vi "cblas ztrsm.vi"(0 "A":T2, 1 "x":T2, 3 "alpha":cdb=1.0+0.0i, 5 "order":T5=101 items=["CblasRowMajor"=101, "CblasColMajor"=102], 6 "transA":T6=111 items=["CblasNoTrans"=111, "CblasTrans"=112, "CblasConjTrans "=113], 7 "uplo":T4=121 items=["CblasUpper"=121, "CblasLower"=122], 8 "lda":i32, 9 "m":i32=-1, 10 "ldx":i32, 11 "n":i32=-1, 12 "diag":T3=131 items=["CblasNonUnit"=131, "CblasUnit"=132], 13 "side":T1=141 items=["CblasLeft"=141, "CblasRight"=142]) -> (14 "ztrsm":T2, 19 "error":i32)   [LabVIEW 2017, in "NI_AALBLAS.lvlib"]
doc: "Operates on matrix <B>A</B> using the operation you select and solves one of the following linear equations for <B>trsm</B>: op(<B>A</B>)*<B>trsm</B> = <B>alpha</B>*<B>X</B> or <B>trsm</B>*op(<B>A</B>) = <B>alpha</B>*<B>X</B>. The data types you wire to <B>A</B> and <B>X</B> determine the polymorphic instance to use."
uses:
  <vilib>/Analysis/NI_AALBLAS.lvlib
  <vilib>/Analysis/Matrix/Datatypes/ComplexMatrix.ctl
  <vilib>/Analysis/BLAS.llb/Operation_Transpose.ctl
  <vilib>/Analysis/BLAS.llb/Order.ctl
  <vilib>/Analysis/BLAS.llb/UpLo.ctl
  <vilib>/Analysis/BLAS.llb/Diag.ctl
  <vilib>/Analysis/BLAS.llb/Side.ctl
  <resource>/lvblas.dll
  <vilib>/Analysis/Matrix/NI_Matrix.lvlib
panel:
  # "void cblas_ztrsm(order, side, uplo, transA, diag, m, n, *alpha, *A, lda, *X, ldx)"
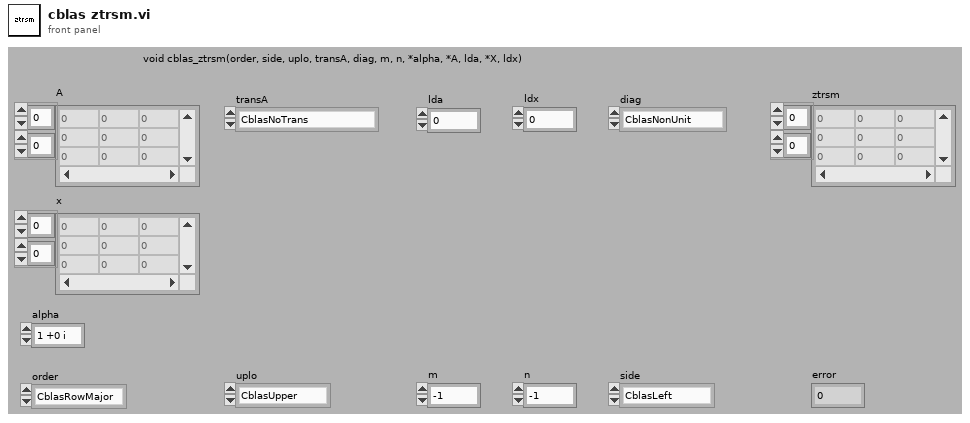
[diagram p1: front panel]
types:
  T1 = typedef "NI_AALBLAS.lvlib/Side.ctl" = i32
  T2 = typedef "NI_Matrix.lvlib/ComplexMatrix.ctl" = cdb[][]
  T3 = typedef "NI_AALBLAS.lvlib/Diag.ctl" = i32
  T4 = typedef "NI_AALBLAS.lvlib/UpLo.ctl" = i32
  T5 = typedef "NI_AALBLAS.lvlib/Order.ctl" = i32
  T6 = typedef "NI_AALBLAS.lvlib/Operation_Transpose.ctl" = i32
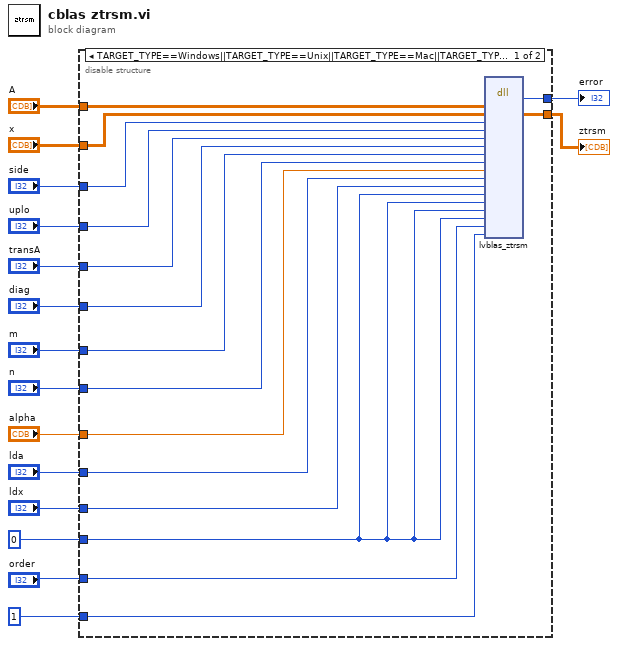
[diagram p0: block diagram]
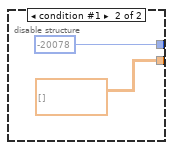
[diagram p2: hidden frame]
diagram:
  n1 = disable-structure shown="TARGET_TYPE==Windows||TARGET_TYPE==Unix||TARGET_TYPE==Mac||TARGET_TYPE==RT" {
    disable-tunnel: "A" -> [w32 _]
    disable-tunnel: [w31 -20078 ("error")] -> w15
    disable-tunnel: 0 -> [w23 _]
    disable-tunnel: [w30 T2 [] ("Complex Matrix")] -> w7
    disable-tunnel: "transA" -> [w26 _]
    disable-tunnel: "uplo" -> [w27 _]
    disable-tunnel: "diag" -> [w25 _]
    disable-tunnel: "x" -> [w29 _]
    disable-tunnel: "side" -> [w28 _]
    disable-tunnel: "alpha" -> [w24 _]
    disable-tunnel: "order" -> [w22 _]
    disable-tunnel: "m" -> [w21 _]
    disable-tunnel: "n" -> [w20 _]
    disable-tunnel: "lda" -> [w19 _]
    disable-tunnel: "ldx" -> [w18 _]
    disable-tunnel: 1 -> [w17 _]
    frame condition #0 (active) {
      n2 = dll-call lib="e:/builds/penguin/labview/branches/2017/dev/dist/resource/lvblas.*" fn="lvblas_ztrsm" ("CBLAS.dll:MtrxxVectH")("a"=w32, "x"=w29, "side"=w28, "uplo"=w27, "OpA"=w26, "diag"=w25, "m"=w21, "n"=w20, "alpha"=w24, "lda"=w19, "ldx"=w18, "startARow"=w23, "startACol"=w23, "startXRow"=w23, "startXCol"=w23, "order"=w22, "check"=w17) -> ("error"=w31:i32, "x"=w30:T2)  [unwired: 19 in, 2 out]
    }
    frame condition #1 {
    }
  }
  "ztrsm" <- w7
  "error" <- w15
